vi "WallFollow.vi"(7 "Inhibit":bool, 8 "HowAmI? Clean":cluster{"T":dbl, "Battery":dbl, "Temp":dbl}, 9 "WhatAroundMe? Clean":cluster{"T":dbl, "Range":dbl, "Bearing":dbl}[](array[cluster]), 10 "WhereAmI? Clean":T2, 11 "Velocity":dbl) -> (0 "SupressOut":dbl, 2 "ActCommand":dbl[](array[numeric]), 4 "InhibitOut":bool)   [LabVIEW 2011]
doc: "This subVI executes a wall folowing Midbrain behaviors. Its inputs are the outputs of the three SENSE processes, the overall velocity requested of the robot, a suppression value from another co-brahvior and an inhibit signal to turn the behavior off. The outputs are a 90 element steering array, a suppression value to diminish the output of co-behaviors and an inhibit output to shut off otehr behaviors.\n\nIt is designed to work with a 90 element behavior arbiter."
panel:
  out "Waveform Chart":dbl(graph)
  out "steer":dbl format="%.2f"
  out "Range":dbl
  in  "PID gains":T1={"proportional gain (Kc)"=20.0, "integral time (Ti, min)"=0.008, "derivative time (Td, min)"=0.001} {"derivative time (Td, min)" format="%.3f"; "integral time (Ti, min)" format="%.3f"; "proportional gain (Kc)" format="%.3f"}
  # "This VI contains a wall following behavior at the Midbrain level"
  # "0.5"
  # "0"
  # "35"
  # "0"
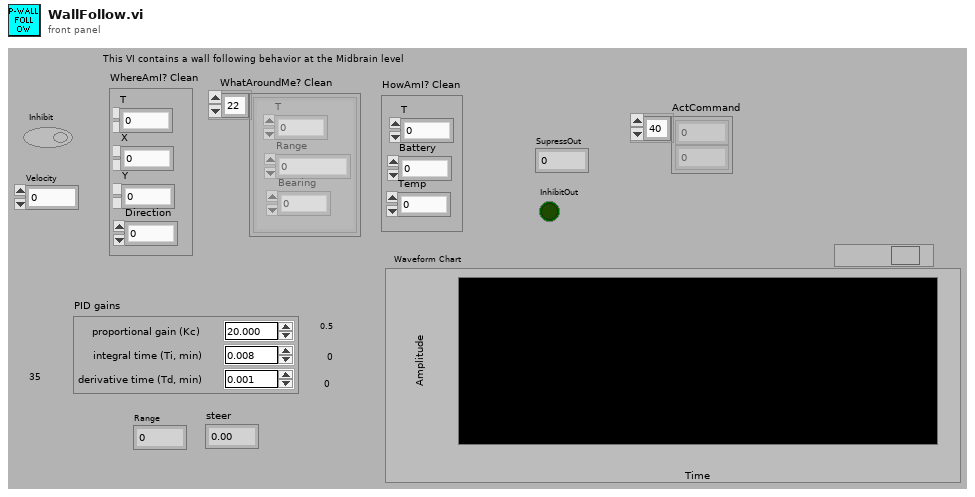
[diagram p1: front panel]
types:
  T1 = cluster{"proportional gain (Kc)":dbl, "integral time (Ti, min)":dbl, "derivative time (Td, min)":dbl}
  T2 = cluster{"T":dbl, "X":dbl, "Y":dbl, "Direction":dbl}
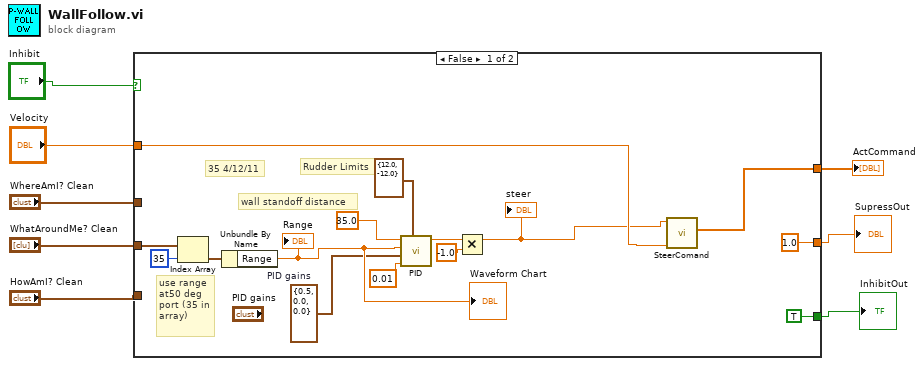
[diagram p0: block diagram]
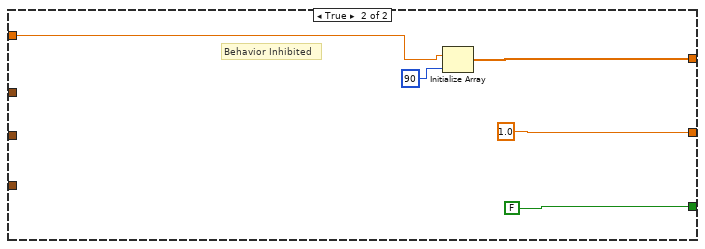
[diagram p2: hidden frame]
diagram:
  n1 = case shown="False" "Inhibit" {
    tunnel: "Velocity" -> [w19 w24]
    tunnel: "WhatAroundMe? Clean" -> [w21 _]
    tunnel: "WhereAmI? Clean" -> [_ _]
    tunnel: "HowAmI? Clean" -> [_ _]
    tunnel: [w18 w26] -> w2
    tunnel: [1.0 ("SupressOut") 1.0 ("SupressOut")] -> w3
    tunnel: [TRUE ("InhibitOut") FALSE ("InhibitOut")] -> w1
    frame False {
      w9 = T1 {"proportional gain (Kc)"=0.5, "integral time (Ti, min)"=0.0, "derivative time (Td, min)"=0.0}  # PID gains
      # "35 4/12/11"
      # "Rudder Limits"
      # "wall standoff distance"
      # "use range \nat50 deg\nport (35 in\narray)"
      n2 = Index Array "Index Array"(array=w21, index=35) -> (element=w20:cluster{"T":dbl, "Range":dbl, "Bearing":dbl})
      n3 = Unbundle By Name(w20) -> ("Range"=w14:dbl)
      "Range" <- w14
      "Waveform Chart" <- w14
      n4 = call "PID.vi"("Range"=cluster{"output high":dbl, "output low":dbl} {"output high"=12.0, "output low"=-12.0} ("output range"), "dt (s)"=0.01, "Control Gains"=w9, "Process Variable"=w14, "Setpoint"=35.0 ("setpoint")) -> ("Command"=w16:dbl)  [unwired: 6 in]
      n5 = Multiply(x=w16, y=-1.0) -> (x*y=w13:dbl)
      "steer" <- w13
      n6 = call "SteerComand.vi"("Speed"=w19, "SteeringAngle"=w13) -> ("ManualActCommand"=w18:dbl[])  [unwired: 9 in]
    }
    frame True {
      # "Behavior Inhibited"
      n7 = Initialize Array "Initialize Array"(w24, 90 ("dimension size")) -> (w26:dbl[])
    }
  }
  "ActCommand" <- w2
  "SupressOut" <- w3
  "InhibitOut" <- w1
